vi "SetStringInfo.vi"(0 "reference":refnum<class "ChoiceNode.lvclass">, 1 "State":string, 2 "Action":string, 5 "error in (no error)":errorcluster) -> (14 "reference out":refnum<class "ChoiceNode.lvclass">, 19 "error out":errorcluster)   [LabVIEW 2012, in "ChoiceNode.lvclass"]
uses:
  <resource>/Framework/Providers/Open_GDS/UML/ChoiceNode_class/ChoiceNode.lvclass
  <resource>/Framework/Providers/Open_GDS/UML/MultiLineString_class/MultiLineString.lvclass
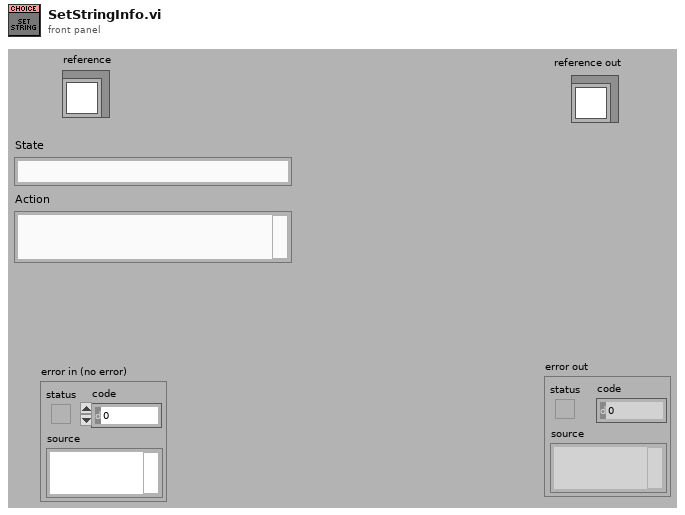
[diagram p1: front panel]
types:
  T1 = typedef "ChoiceNode.lvclass/ObjectAttributes.ctl" = cluster{"Base class":T2, "Text":refnum<class "MultiLineString.lvclass">, "DEFAULT_WIDTH":i32, "DEFAULT_HEIGHT":i32}
  T2 = typedef "RectangularNode.lvclass/ObjectAttributes.ctl" = cluster{"Base class":T3, "bounds":T4}
  T3 = typedef "AbstractNode.lvclass/ObjectAttributes.ctl" = cluster{"parent":refnum<class "AbstractNode.lvclass">, "children":refnum<class "AbstractNode.lvclass">[], "Hidden":bool}
  T4 = typedef "Rectangle Rectangle2D.ctl" = cluster{"x":dbl, "y":dbl, "width":dbl, "height":dbl}
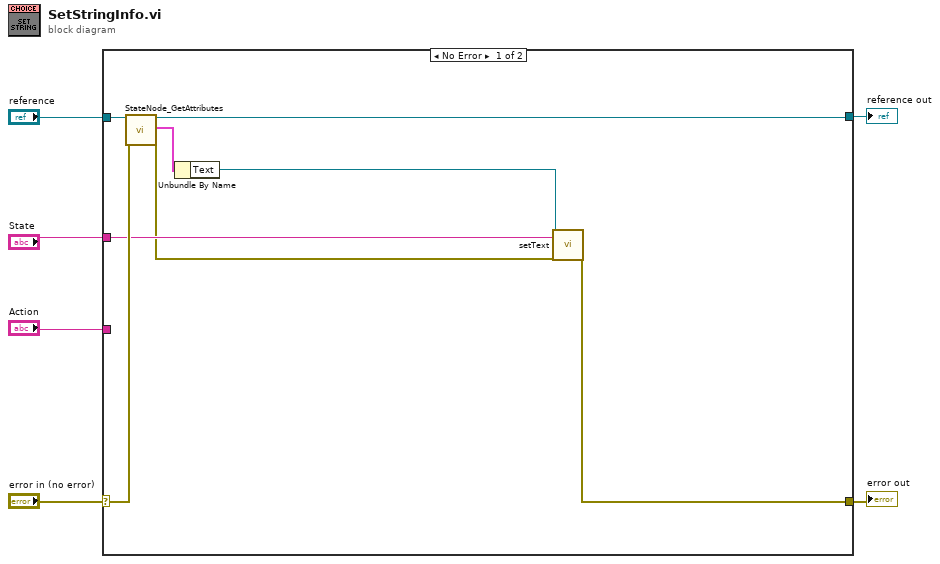
[diagram p0: block diagram]
diagram:
  n1 = case shown="No Error" "error in (no error)" {
    selector: "error in (no error)" -> [w14 w15]
    tunnel: "reference" -> [w13 w16]
    tunnel: [w9 w15] -> w4
    tunnel: [w12 w16] -> w3
    tunnel: "State" -> [w8 _]
    tunnel: "Action" -> [_ _]
    frame No Error {
      n2 = call <resource>:"StateNode_GetAttributes.vi"("reference in"=w13, "error in (no error)"=w14) -> ("reference out"=w12:refnum<class "ChoiceNode.lvclass">, "Attributes"=w10:T1, "error out"=w7:errorcluster)  [unwired: 15 out]
      n3 = Unbundle By Name(w10) -> ("Text"=w11:refnum<class "MultiLineString.lvclass">)
      n4 = call-dynamic "setText.vi"("reference"=w11, "text"=w8, "error in (no error)"=w7) -> ("error out"=w9:errorcluster)  [unwired: 16 out]
    }
    frame Error {
    }
  }
  "reference out" <- w3
  "error out" <- w4
